vi "write speedline data to file.vi"(11 "makeSpeedlinesData in":T1) -> (3 "makeSpeedlinesData out":T1)   [LabVIEW 2018]
uses:
  make speedlines UI data.ctl
types:
  T1 = typedef "make speedlines UI data.ctl" = cluster{"folder":path, "PR Channel":u16, "Massflow Channel":u16, "speedlineCount":u16, "massFlowData":dbl[], "PRdata":dbl[], "progress":refnum<vi>, "PR":refnum<vi>, "massflow":refnum<vi>, "speedlineFileRef":refnum<file>, "speedlineFile":path, "speedlines":cluster{"mDot":dbl[], "PR":dbl[]}[]}
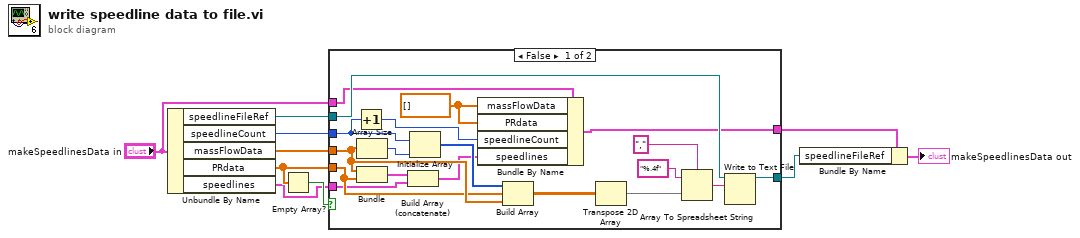
[diagram p0: block diagram]
diagram:
  n1 = Unbundle By Name("makeSpeedlinesData in") -> ("speedlineFileRef"=w9:refnum<file>, "speedlineCount"=w8:u16, "massFlowData"=w7:dbl[], "PRdata"=w5:dbl[], "speedlines"=w1:cluster{"mDot":dbl[], "PR":dbl[]}[])
  n2 = Empty Array?(array=w5) -> (empty?=w4:bool)
  n3 = case shown="False" w4 {
    tunnel: w9 -> [w29 w31]
    tunnel: w5 -> [w14 _]
    tunnel: w8 -> [w18 _]
    tunnel: w7 -> [w15 _]
    tunnel: [w22 w31] -> w6
    tunnel: "makeSpeedlinesData in" -> [w21 w30]
    tunnel: [w19 w30] -> w2
    tunnel: w1 -> [w13 _]
    frame False {
      w20 = dbl[] [] ("massFlowData")
      n4 = Increment(x=w18) -> (x+1=w17:u16)
      n5 = Array Size(array=w15) -> (size(s)=w24:i32)
      n6 = Bundle("massFlowData"=w15, "PRdata"=w14) -> (w12:cluster{"massFlowData":dbl[], "PRdata":dbl[]})  [unwired: 1 in]
      n7 = Build Array (concatenate)(w12, w13) -> (w11:cluster{"mDot":dbl[], "PR":dbl[]}[])
      n8 = Initialize Array(w18, w24) -> (w23:u16[])
      n9 = Bundle By Name(cluster=w21, "massFlowData"=w20, "PRdata"=w20, "speedlineCount"=w17, "speedlines"=w11) -> (w19:T1)
      n10 = Build Array(w23, w14, w15) -> (w28:dbl[][])
      n11 = Transpose 2D Array(2D array=w28) -> (transposed array=w16:dbl[][])
      n12 = Array To Spreadsheet String(delimiter (Tab)=",", array=w16, 3:"%.4f" ("format string")) -> (spreadsheet string=w25:string)
      n13 = Write to Text File(file (use dialog)=w29, text=w25) -> (refnum out=w22:refnum<file>)  [unwired: 2 in, 2 out]
    }
    frame True {
    }
  }
  n14 = Bundle By Name(cluster=w2, "speedlineFileRef"=w6) -> (→"makeSpeedlinesData out":T1)
